vi "Network stream harness.vi"() -> ()   [LabVIEW 2018]
uses:
  RT/Type Defs/RT Status.ctl
  RT/Type Defs/generic incident.ctl
panel:
  out "RT status":T1
  out "data":bool
  out "command":bool
  out "error":bool
  out "data out":sgl[][](array[numeric])
  in  "STOP":bool
  # "Timeouts:"
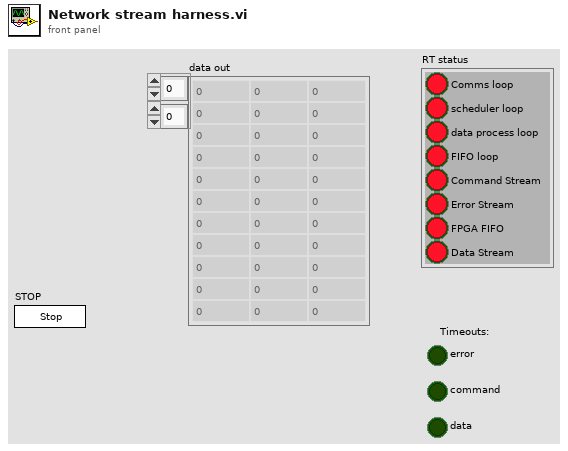
[diagram p1: front panel]
types:
  T1 = typedef "RT Status.ctl" = cluster{"Comms loop":bool, "scheduler loop":bool, "data process loop":bool, "FIFO loop":bool, "Command Stream":bool, "Error Stream":bool, "FPGA FIFO":bool, "Data Stream":bool}
  T2 = typedef "generic incident.ctl" = cluster{"timestamp":timestamp, "type":string, "Variant":variant}
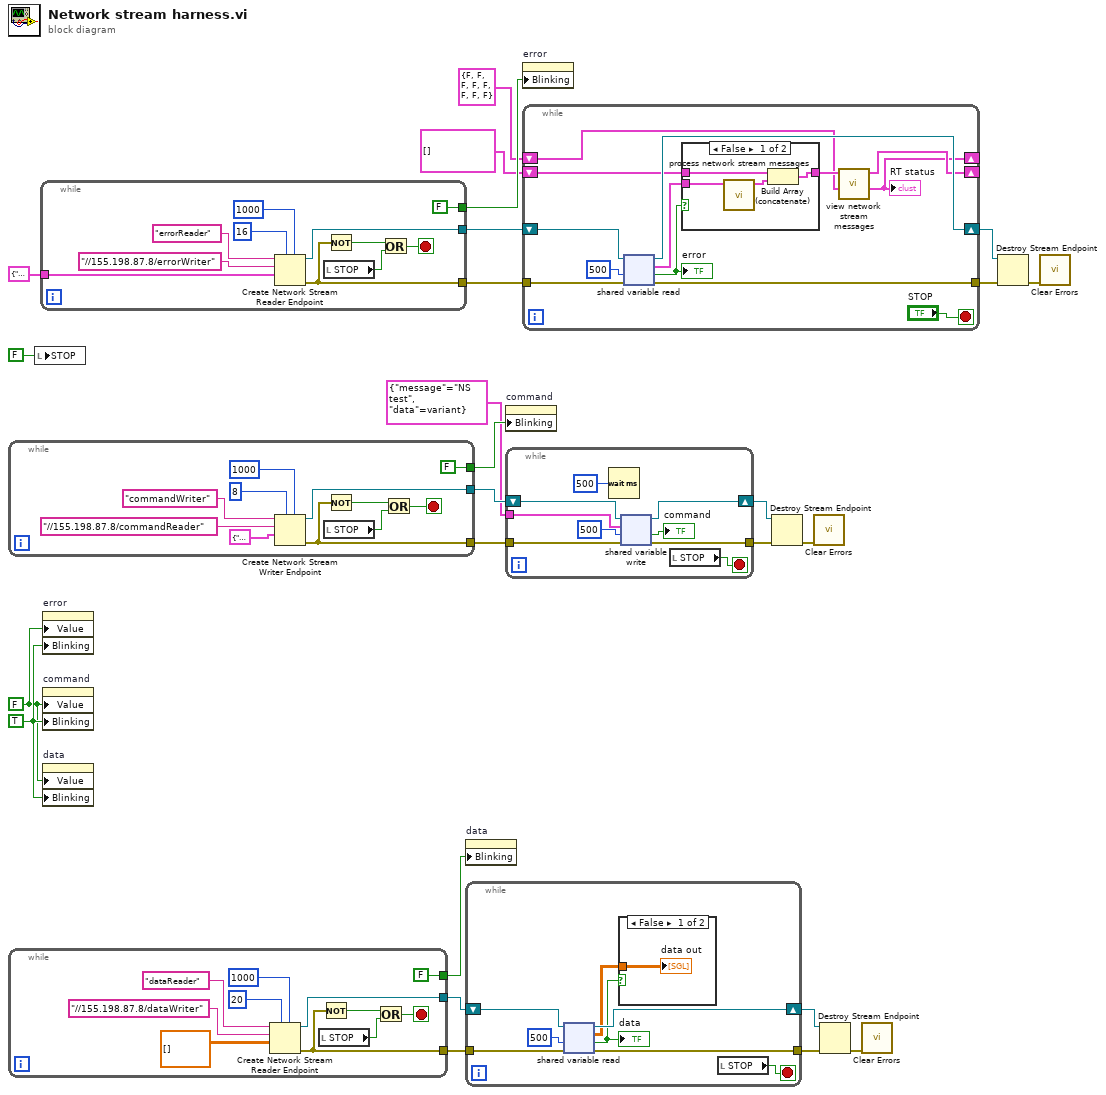
[diagram p0: block diagram]
diagram:
  w5 = FALSE ("Blinking")
  w12 = TRUE ("Blinking")
  n1 = while {
    tunnel: [w32] -> w23
    tunnel: [w29] -> w22
    tunnel: [FALSE ("Blinking")] -> w10
    stop <- w26 stop-if-true
    n2 = Create Network Stream Writer Endpoint(5:1000 ("timeout in ms (-1)"), 7:8 ("reader buffer size"), 9:cluster{"message":string, "data":variant} {"message"="", "data"=variant}, 10:"//155.198.87.8/commandReader" ("writer url"), 11:"commandWriter" ("reader name")) -> (0:w29:errorcluster, 3:w32:refnum<k21>)  [unwired: 2 in]
    n3 = local read "STOP"() -> (w27:bool)
    n4 = Not(x=w29) -> (.not. x?=w28:bool)
    n5 = Or(x=w28, y=w27) -> (x .or. y?=w26:bool)
  }
  n6 = while {
    tunnel: [w43] -> w15
    tunnel: [w39] -> w14
    tunnel: [FALSE ("Blinking")] -> w11
    stop <- w37 stop-if-true
    n7 = Create Network Stream Reader Endpoint(5:1000 ("timeout in ms (-1)"), 7:20 ("reader buffer size"), 9:sgl[][] [], 10:"//155.198.87.8/dataWriter" ("writer url"), 11:"dataReader" ("reader name")) -> (0:w39:errorcluster, 3:w43:refnum<k21>)  [unwired: 2 in]
    n8 = local read "STOP"() -> (w38:bool)
    n9 = Not(x=w39) -> (.not. x?=w40:bool)
    n10 = Or(x=w40, y=w38) -> (x .or. y?=w37:bool)
  }
  n11 = local write "STOP"(FALSE ("STOP")) -> ()
  n12 = while {
    tunnel: cluster{"message":string, "data":variant} {"message"="", "data"=variant} -> [w58]
    tunnel: [w54] -> w20
    tunnel: [w48] -> w18
    tunnel: [FALSE ("Blinking")] -> w13
    stop <- w50 stop-if-true
    n13 = Create Network Stream Reader Endpoint(5:1000 ("timeout in ms (-1)"), 7:16 ("reader buffer size"), 9:w58, 10:"//155.198.87.8/errorWriter" ("writer url"), 11:"errorReader" ("reader name")) -> (0:w48:errorcluster, 3:w54:refnum<k21>)  [unwired: 2 in]
    n14 = local read "STOP"() -> (w49:bool)
    n15 = Not(x=w48) -> (.not. x?=w51:bool)
    n16 = Or(x=w51, y=w49) -> (x .or. y?=w50:bool)
  }
  n17 = property on="error" class="Bool (strict)"("Value"=w5, "Blinking"=w12) -> ()  [unwired: 2 in, 2 out]
  n18 = property on="command" class="Bool (strict)"("Value"=w5, "Blinking"=w12) -> ()  [unwired: 2 in, 2 out]
  n19 = property on="data" class="Bool (strict)"("Value"=w5, "Blinking"=w12) -> ()  [unwired: 2 in, 2 out]
  n20 = property on="data" class="Bool (strict)"("Blinking"=w11) -> ()  [unwired: 2 in, 2 out]
  n21 = while {
    tunnel: w14 -> [w64]
    shift-right: [w63] -> w16
    shift-left: w15 -> [w65]
    tunnel: [w62] -> w17
    stop <- w66 stop-if-true
    n22 = shared-variable-read(w65, w64, 500 ("timeout ms (-1)")) -> (w63:refnum<k21>, w62:errorcluster, w59:bool, w61:sgl[][])
    "data" <- w59
    n23 = case shown="False" w59 {
      tunnel: w61 -> [w67 _]
      frame False {
        "data out" <- w67
      }
      frame True {
      }
    }
    n24 = local read "STOP"() -> (w66:bool)
  }
  n25 = property on="command" class="Bool (strict)"("Blinking"=w10) -> ()  [unwired: 2 in, 2 out]
  n26 = while {
    shift-right: [w73] -> w25
    shift-left: w23 -> [w74]
    tunnel: w22 -> [w72]
    tunnel: [w71] -> w24
    tunnel: cluster{"message":string, "data":variant} {"message"="NS test", "data"=variant} -> [w68]
    stop <- w75 stop-if-true
    n27 = Wait (ms)(milliseconds to wait=u32 500) -> ()  [unwired: 1 out]
    n28 = shared-variable-write(w74, w72, w68, 500 ("timeout ms (-1)")) -> (w73:refnum<k21>, w71:errorcluster, →"command":bool)
    n29 = local read "STOP"() -> (w75:bool)
  }
  n30 = property on="error" class="Bool (strict)"("Blinking"=w13) -> ()  [unwired: 2 in, 2 out]
  n31 = while {
    tunnel: w18 -> [w87]
    shift-right: [w86] -> w21
    shift-left: w20 -> [w88]
    tunnel: [w85] -> w19
    shift-right: [w79] -> _
    shift-left: T2[] [] ("Array") -> [w81]
    shift-right: [w78] -> _
    shift-left: T1 {"Comms loop"=FALSE, "scheduler loop"=FALSE, "data process loop"=FALSE, "FIFO loop"=FALSE, "Command Stream"=FALSE, "Error Stream"=FALSE, "FPGA FIFO"=FALSE, "Data Stream"=FALSE} ("RT status") -> [w77]
    stop <- "STOP" stop-if-true
    n32 = shared-variable-read(w88, w87, 500 ("timeout ms (-1)")) -> (w86:refnum<k21>, w85:errorcluster, w82:bool, w84:cluster{"message":string, "data":variant})
    "error" <- w82
    n33 = case shown="False" w82 {
      tunnel: w84 -> [w93 _]
      tunnel: w81 -> [w92 w94]
      tunnel: [w90 w94] -> w80
      frame False {
        n34 = call "process network stream messages.vi"("Cluster"=w93) -> ("data"=w91:T2)  [unwired: 9 in, 1 out]
        n35 = Build Array (concatenate)(w92, w91) -> (w90:T2[])
      }
      frame True {
      }
    }
    n36 = call "view network stream messages.vi"("RT status"=w77, "Array"=w80) -> ("RT status"=w78:T1, "Array out"=w79:T2[])  [unwired: 8 in]
    "RT status" <- w78
  }
  n37 = Destroy Stream Endpoint(8:w24, 11:w25) -> (0:w7:errorcluster)
  n38 = call <vilib>:"Clear Errors.vi"("error in (no error)"=w7) -> ()  [unwired: 5 in, 2 out]
  n39 = Destroy Stream Endpoint(8:w17, 11:w16) -> (0:w6:errorcluster)
  n40 = call <vilib>:"Clear Errors.vi"("error in (no error)"=w6) -> ()  [unwired: 5 in, 2 out]
  n41 = Destroy Stream Endpoint(8:w19, 11:w21) -> (0:w8:errorcluster)
  n42 = call <vilib>:"Clear Errors.vi"("error in (no error)"=w8) -> ()  [unwired: 5 in, 2 out]
